vi "Data_Base_logging.vi"() -> (1 "Logging On?":bool, 2 "Close Loop with Pitot?":bool, 3 "Rig Name":string="Run EnFlo Hub.vi", 4 "DB Setup files":string[](array[string])=["EnFlo Tun DB setup.xls", "A Tunnel DB setup.xls", "D Tunnel DB setup.xls", "Aero Tunnel DB setup.xls"])   [LabVIEW 2010]
uses:
  Controls/Server_Comms.ctl
  Globals/Preference_global.vi
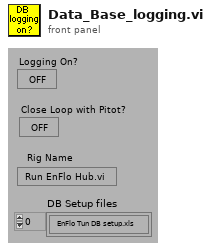
[diagram p1: front panel]
types:
  T1 = typedef "Server_Comms.ctl" = enum16{"Server Link Healthy", "Do Not Link To Server"}
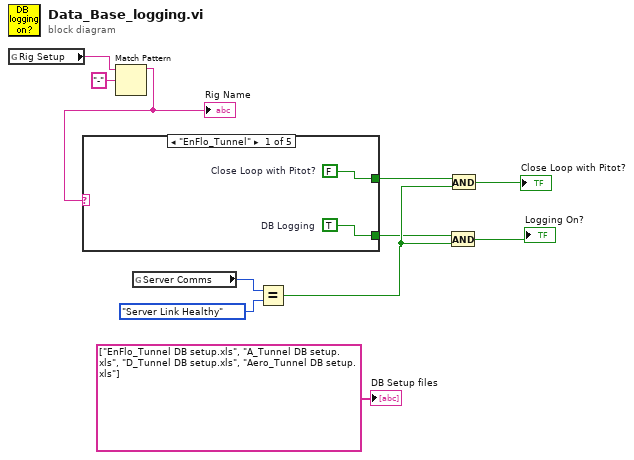
[diagram p0: block diagram]
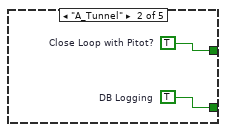
[diagram p2: hidden frame]
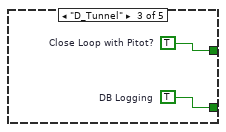
[diagram p3: hidden frame]
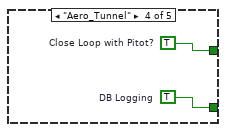
[diagram p4: hidden frame]
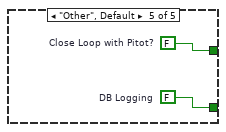
[diagram p5: hidden frame]
diagram:
  n1 = global read "Preference_global.vi" "Rig Setup"() -> (w3:string)
  n2 = Match Pattern(string=w3, regular expression="-") -> (before substring=w1:string)  [unwired: 4 out]
  "Rig Name" <- w1
  n3 = case shown="\"EnFlo_Tunnel\"" w1 {
    tunnel: [w13 w15 w17 w19 w21] -> w5
    tunnel: [w12 w14 w16 w18 w20] -> w4
    frame "EnFlo_Tunnel" {
      w12 = TRUE  # DB Logging
      w13 = FALSE  # Close Loop with Pitot?
    }
    frame "A_Tunnel" {
      w14 = TRUE  # DB Logging
      w15 = TRUE  # Close Loop with Pitot?
    }
    frame "D_Tunnel" {
      w16 = TRUE  # DB Logging
      w17 = TRUE  # Close Loop with Pitot?
    }
    frame "Aero_Tunnel" {
      w18 = TRUE  # DB Logging
      w19 = TRUE  # Close Loop with Pitot?
    }
    frame "Other", Default {
      w20 = FALSE  # DB Logging
      w21 = FALSE  # Close Loop with Pitot?
    }
  }
  n4 = global read "Preference_global.vi" "Server Comms"() -> (w10:T1)
  n5 = Equal?(x=w10, y=Server_Comms."Server Link Healthy" ("Server Comms")) -> (x = y?=w6:bool)
  n6 = And(x=w4, y=w6) -> (x .and. y?=→"Logging On?":bool)
  n7 = And(x=w5, y=w6) -> (x .and. y?=→"Close Loop with Pitot?":bool)
  "DB Setup files" <- string[] ["EnFlo_Tunnel DB setup.xls", "A_Tunnel DB setup.xls", "D_Tunnel DB setup.xls", "Aero_Tunnel DB setup.xls"] ("appended array")
